vi "robot_UDP_Transaction.vi"(11 "connection ID":refnum<k16>) -> (0 "status":bool, 3 "Dashboard Return Data":T1)   [LabVIEW 2011]
uses:
  dashboard_return_data.ctl
  2012vision/Camera State.ctl
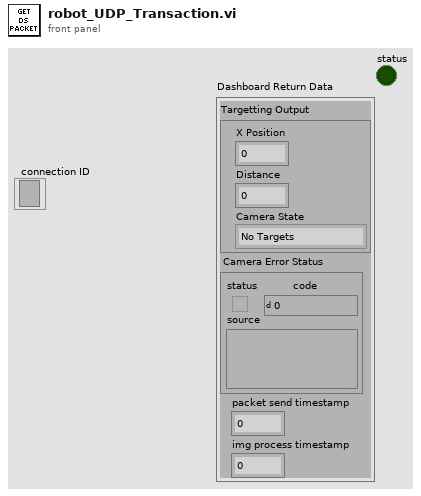
[diagram p1: front panel]
types:
  T1 = typedef "dashboard_return_data.ctl" = cluster{"Targetting Output":cluster{"X Position":dbl, "Distance":dbl, "Camera State":T2}, "Camera Error Status":errorcluster, "packet send timestamp":u32, "img process timestamp":u32}
  T2 = typedef "Camera State.ctl" = enum16{"No Targets", "Low Confidence", "Medium Confidence", "High Confidence", "Camera Error"}
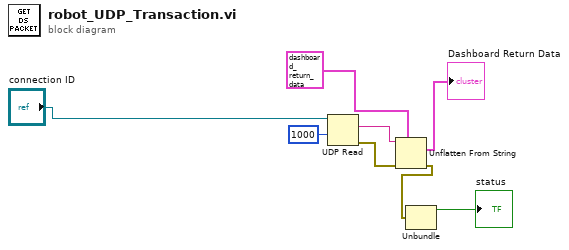
[diagram p0: block diagram]
diagram:
  n1 = UDP Read(connection ID="connection ID", timeout ms (25000)=1000) -> (data out=w8:string, error out=w4:errorcluster)  [unwired: 2 in, 3 out]
  n2 = Unflatten From String(type=T1 {"Targetting Output"={"X Position"=0.0, "Distance"=0.0, "Camera State"=enum."No Targets"}, "Camera Error Status"={"status"=FALSE, "code"=0, "source"=""}, "packet send timestamp"=0, "img process timestamp"=0} ("Dashboard Return Data"), binary string=w8, error in (no error)=w4) -> (value=→"Dashboard Return Data":T1, error out=w3:errorcluster)  [unwired: 2 in, 1 out]
  n3 = Unbundle(w3) -> ("status"=→"status":bool)  [unwired: 2 out]
